vi "EngFormatScaleFactor.vi"(10 "Input Number":ext format="%#.2e") -> (2 "Engineering Format Scale Factor":dbl format="%#.2e")   [LabVIEW 2014]
panel:
  # "This program extracts the engineering format scale value from the input number."
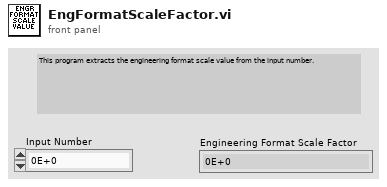
[diagram p1: front panel]
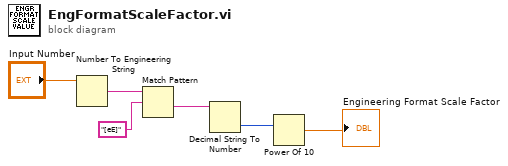
[diagram p0: block diagram]
diagram:
  n1 = Number To Engineering String(4:"Input Number") -> (0:w5:string)  [unwired: 3 out]
  n2 = Match Pattern(string=w5, regular expression="[eE]") -> (after substring=w4:string)  [unwired: 4 out]
  n3 = Decimal String To Number(string=w4) -> (number=w2:i32)  [unwired: 3 out]
  n4 = Power Of 10(x=w2) -> (10^x=→"Engineering Format Scale Factor":dbl)
